vi "Compute DistanceTo Coral2.vi"(6 "Robot Calibration Cluster":T2={"Camera Height on robot (in)"=34.5, "Camera Angle on the robot (deg)"=28.3, "Camera FOV Top to Bottom View Angle (deg)"=0.946, "Camera FOV Left to Right View Angle (deg)"=26.5, "Target size (in)"=6.5, "Distance to front of bumper (in)"=9.75, "Focal Length (mm)"=10.0, "Yaw Slope"=9.75, "Yaw Offset"=10.0} {"Yaw Offset" format="%#_13g"; "Yaw Slope" format="%#_13g"; "Camera FOV Left to Right View Angle (deg)" format="%#_13g"; "Focal Length (mm)" format="%#_13g"; "Distance to front of bumper (in)" format="%#_13g"; "Target size (in)" format="%#_13g"; "Camera FOV Top to Bottom View Angle (deg)" format="%#_13g"; "Camera Angle on the robot (deg)" format="%#_13g"; "Camera Height on robot (in)" format="%#_13g"}, 8 "results 2":T1, 11 "Image Src":T3) -> (0 "results out":T1, 2 "Offset Angle":dbl=569.258018632146, 3 "Image Dst Out":T3, 4 "Distance from target (in)":dbl=116.40675998176638 format="%.2f")   [LabVIEW 2023]
doc: "Using the camera lens information and the real world size of the target, use trig and ratios to determine the distance to the target. Also returns the location relative to the image center in a (-1 , 1) coordinate system that may be useful for steering the robot."
uses:
  <vilib>/vision/Image Controls.llb/IMAQ Image.ctl
  April Tags/Camera Info.ctl
  Target Fields.ctl
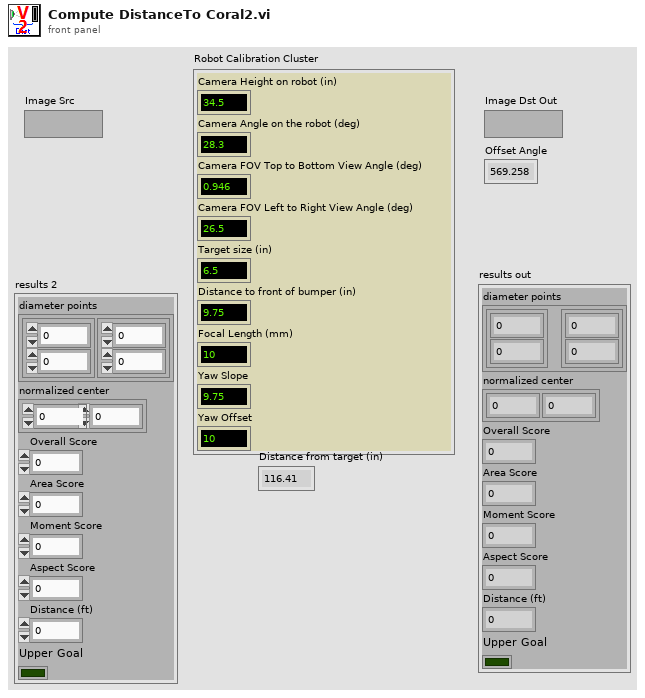
[diagram p1: front panel]
types:
  T1 = typedef "Target Fields.ctl" = cluster{"diameter points":cluster{"first point":cluster{"x":dbl, "y":dbl}, "projected point":cluster{"x":dbl, "y":dbl}}, "normalized center":cluster{"x":dbl, "y":dbl}, "Overall Score":dbl, "Area Score":dbl, "Moment Score":dbl, "Aspect Score":dbl, "Distance (ft)":dbl, "Upper Goal":bool}
  T2 = typedef "Camera Info.ctl" = cluster{"Camera Height on robot (in)":dbl, "Camera Angle on the robot (deg)":dbl, "Camera FOV Top to Bottom View Angle (deg)":dbl, "Camera FOV Left to Right View Angle (deg)":dbl, "Target size (in)":dbl, "Distance to front of bumper (in)":dbl, "Focal Length (mm)":dbl, "Yaw Slope":dbl, "Yaw Offset":dbl}
  T3 = typedef "IMAQ Image.ctl" = refnum<image>
  T4 = cluster{"first point":cluster{"x":dbl, "y":dbl}, "projected point":cluster{"x":dbl, "y":dbl}}
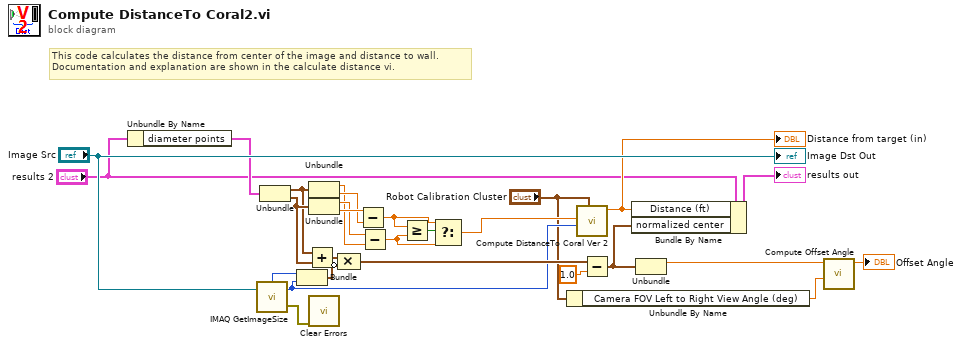
[diagram p0: block diagram]
diagram:
  # "This code calculates the distance from center of the image and distance to wall.\nDocumentation and explanation are shown in the calculate distance vi."
  n1 = Unbundle By Name("results 2") -> ("diameter points"=w11:T4)
  n2 = call "IMAQ GetImageSize"("Image"="Image Src") -> ("Y Resolution"=w18:i32, "X Resolution"=w19:i32, "error out"=w27:errorcluster)  [unwired: 3 in]
  n3 = Unbundle(w11) -> ("first point"=w14:cluster{"x":dbl, "y":dbl}, "projected point"=w17:cluster{"x":dbl, "y":dbl})
  n4 = Bundle("X Resolution"=w19, "Y Resolution"=w18) -> (w13:cluster{"X Resolution":i32, "Y Resolution":i32})  [unwired: 1 in]
  n5 = Add(x=w14, y=w17) -> (x+y=w24:cluster{"x":dbl, "y":dbl})
  n6 = Unbundle(w14) -> ("x"=w3:dbl, "y"=w15:dbl)
  n7 = Unbundle(w17) -> ("x"=w4:dbl, "y"=w16:dbl)
  n8 = call <vilib>:"Clear Errors.vi"("error in (no error)"=w27) -> ()  [unwired: 5 in, 2 out]
  n9 = Compound Arithmetic op=MULTIPLY(w24, invert w13) -> (w25:cluster{dbl, dbl})
  n10 = Subtract(x=w16, y=w15) -> (x-y=w7:dbl)
  n11 = Subtract(x=w4, y=w3) -> (x-y=w6:dbl)
  n12 = Greater Or Equal?(x=w7, y=w6) -> (x >= y?=w8:bool)
  n13 = Select(t=w7, s=w8, f=w6) -> (s? t:f=w5:dbl)
  n14 = Unbundle By Name("Robot Calibration Cluster") -> ("Camera FOV Left to Right View Angle (deg)"=w1:dbl)
  n15 = call "Compute DistanceTo Coral Ver 2.vi"("Robot Calibration Cluster"="Robot Calibration Cluster", "Screen resolution pixels Height (Ry)"=w18, "Target Vertical pixels bottom - top (pixels)"=w5) -> ("Distance from target (in)"=w12:dbl)  [unwired: 8 in]
  "Distance from target (in)" <- w12
  n16 = Subtract(x=w25, y=1.0) -> (x-y=w22:cluster{dbl, dbl})
  n17 = Bundle By Name(cluster="results 2", "Distance (ft)"=w12, "normalized center"=w22) -> (→"results out":T1)
  n18 = Unbundle(w22) -> (w21:dbl)  [unwired: 1 out]
  n19 = call "Compute Offset Angle.vi"("Field of view"=w1, "Offset Normilized"=w21) -> ("Offset Angle"=→"Offset Angle":dbl)  [unwired: 9 in]
  "Image Dst Out" <- "Image Src"
